vi "Streaming_control.vi"(8 "error in (no error)":errorcluster, 9 "Configuration":cluster{"prompt":bool}, 10 "State":enum16{"Config", "Run", "Monitor", "Stop"}(ring), 11 "Streaming VI Ref in":refnum<vi>) -> (0 "error out":errorcluster, 1 "Current":waveform(dbl), 2 "Voltage":waveform(dbl))   [LabVIEW 2012]
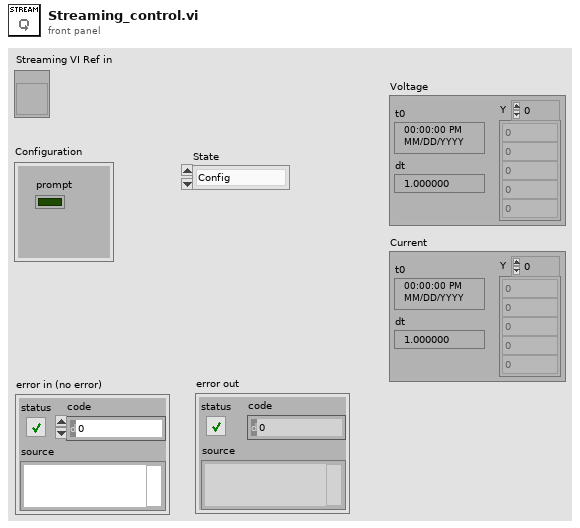
[diagram p1: front panel]
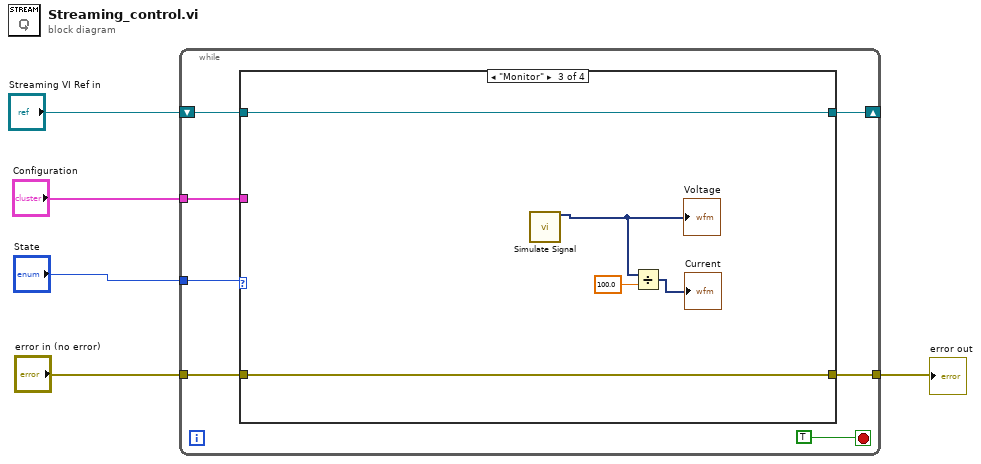
[diagram p0: block diagram]
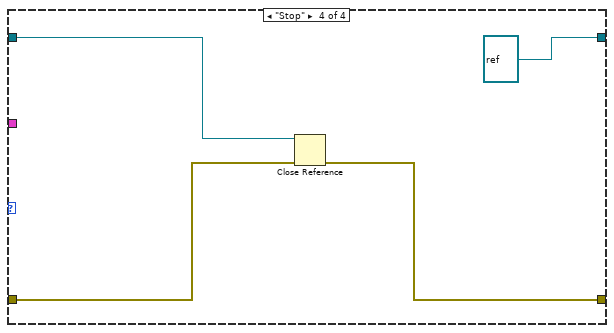
[diagram p4: hidden frame]
diagram:
  n1 = while {
    shift-right: [w9] -> _
    shift-left: "Streaming VI Ref in" -> [w11]
    tunnel: "State" -> [w10]
    tunnel: "Configuration" -> [w8]
    tunnel: "error in (no error)" -> [w7]
    tunnel: [w6] -> w1
    stop <- TRUE ("stop") stop-if-true
    n2 = case shown="\"Monitor\"" w10 {
      tunnel: w11 -> [w14 w16 w21 w25]
      tunnel: [w14 w16 w21 refnum<vi> refnum ("Streaming VI Ref in")] -> w9
      tunnel: w8 -> [_ _ _ _]
      tunnel: w7 -> [w13 w15 w17 w24]
      tunnel: [w13 w15 w17 w23] -> w6
      frame "Config", Default {
      }
      frame "Run" {
      }
      frame "Monitor" {
        n3 = call "Simulate Signal"() -> ("Sine with Uniform Noise"=w20:dynamicdata)  [unwired: 14 in, 1 out]
        "Voltage" <- w20
        n4 = Divide(x=w20, y=100.0) -> (x/y=→"Current":dynamicdata)
      }
      frame "Stop" {
        n5 = Close Reference(reference=w25, error in (no error)=w24) -> (error out=w23:errorcluster)
      }
    }
  }
  "error out" <- w1
